vi "FGV.vi"(6 "Dev Type in":T1, 7 "Dev Type Key":string, 8 "error in (no error)":errorcluster, 9 "Device Types in":T1[](array[typedef]), 10 "Action":T6, 11 "Device Type to return":i32=-1) -> (0 "error out":errorcluster, 1 "Dev Types out":T1[](array[typedef]), 2 "found at index":i32, 3 "added?":bool, 4 "Dev Type out":T1)   [LabVIEW 2013, in "daqio minimal.lvlib"]
doc: "This VI is a functional global variable that stores all relevant daq.io account data locally. \n\nKeeping a local device store helps with managing the device data and improves the performance of the overall system. The daq.io LabVIEW API uses this FGV to track and sync required changes that have to be performed online. This FGV should be updated whenever new channels, tags or event types need to generated. The shipping VIs that implicitly auto-create these channels, tags and events make use of this FGV.\n\nTo conserve the amount of transferred data, you can bypass the FGV and use the low level API Call Functions. Then all potential API errors, such as duplicate keys have to be managed on the client side.\n\nSee the \"Connect Device\" function to learn how this FGV can be used."
uses:
  daqio minimal.lvlib
  _typedefs/daqio-Device-Type-Info-return.ctl
  _typedefs/daqio-Channel-Type-POST-return.ctl
  _typedefs/daqio-Device.ctl
  _typedefs/daqio-Event-Type.ctl
  _typedefs/daqio-Tag-Type-POST-return.ctl
  _typedefs/FGV_commands.ctl
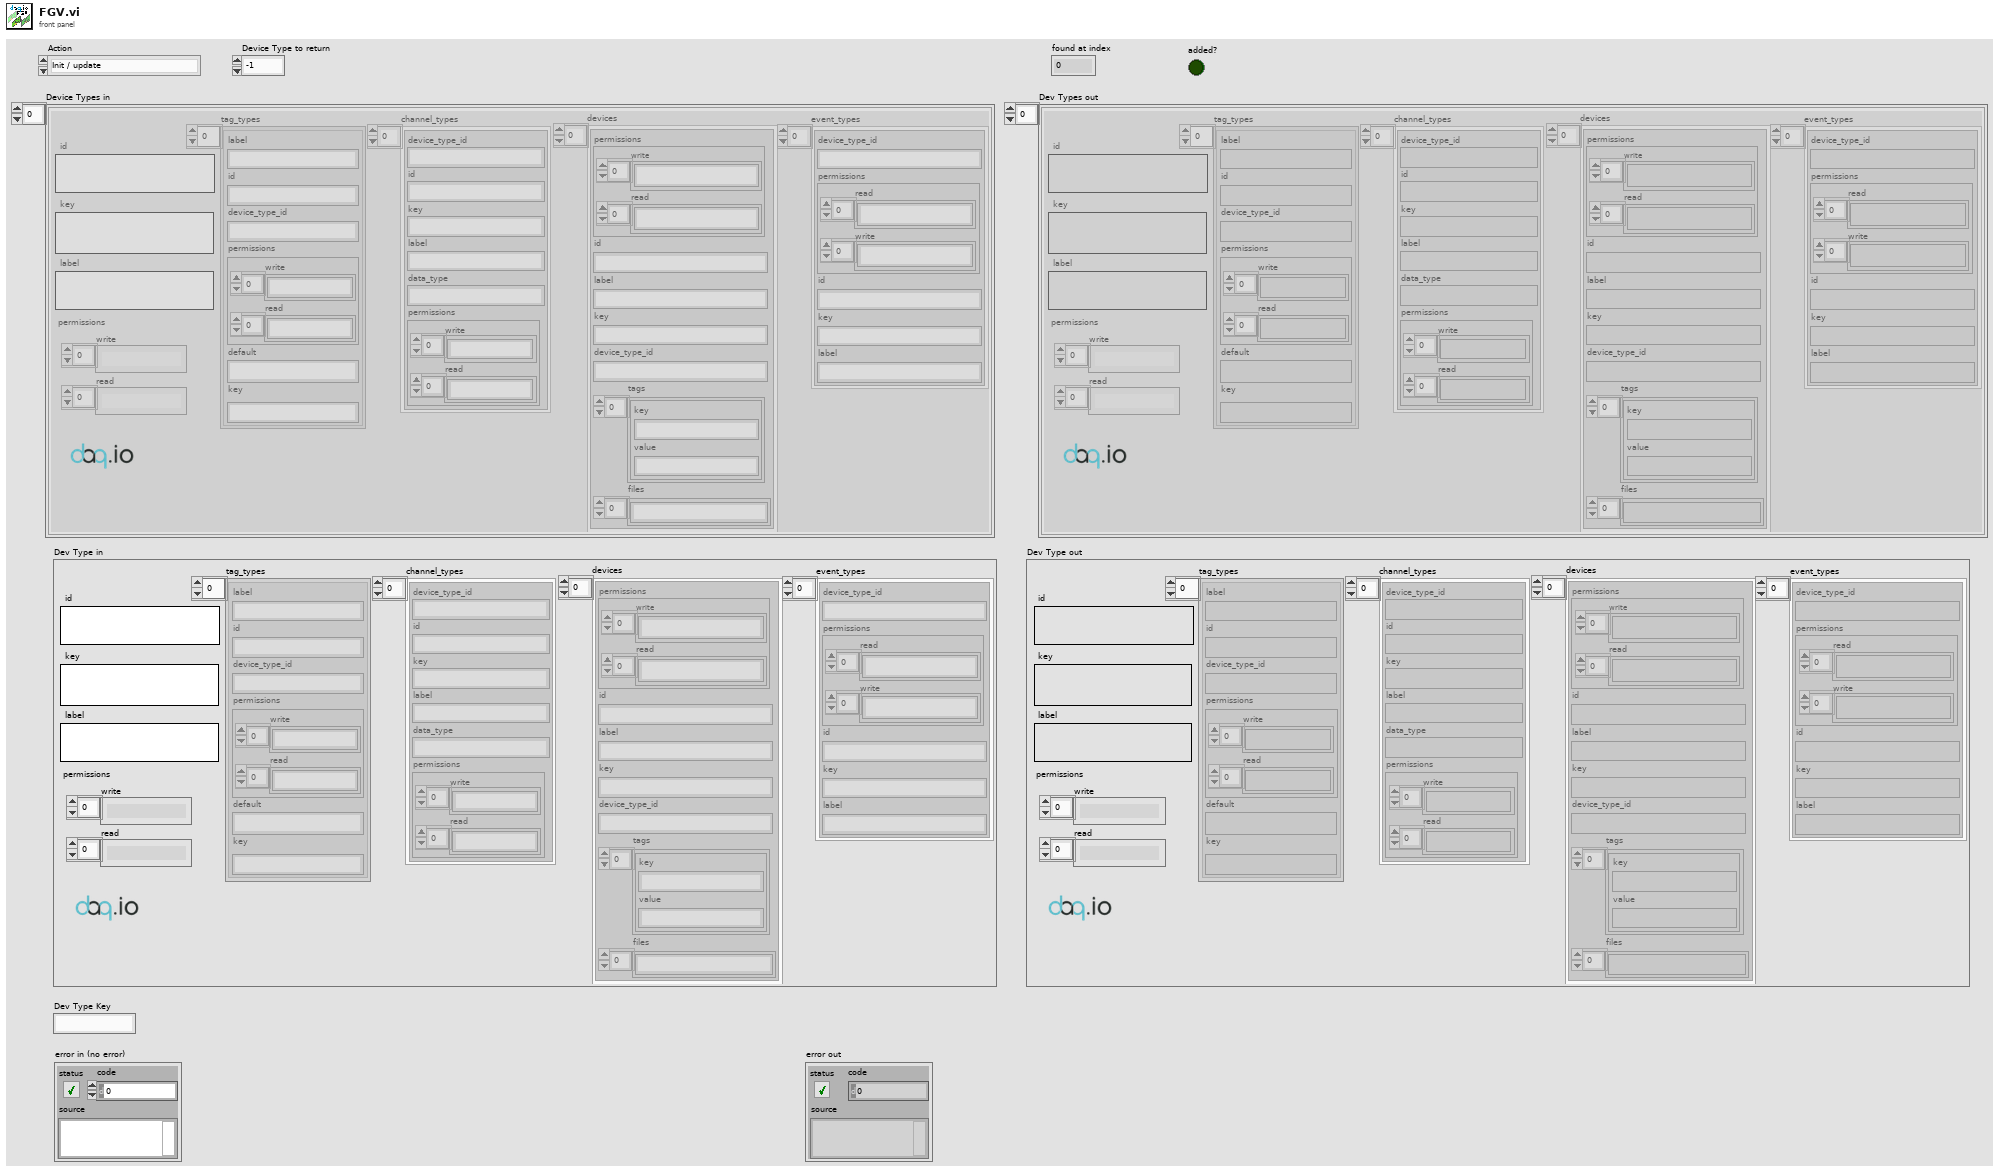
[diagram p1: front panel]
types:
  T1 = typedef "daqio minimal.lvlib/daqio-Device-Type-Info-return.ctl" = cluster{"channel_types":T2[], "devices":T3[], "label":string, "event_types":T4[], "key":string, "tag_types":T5[], "id":string, "permissions":cluster{"write":string[], "read":string[]}}
  T2 = typedef "daqio minimal.lvlib/daqio-Channel-Type-POST-return.ctl" = cluster{"device_type_id":string, "id":string, "key":string, "label":string, "data_type":string, "permissions":cluster{"write":string[], "read":string[]}}
  T3 = typedef "daqio minimal.lvlib/daqio-Device.ctl" = cluster{"permissions":cluster{"write":string[], "read":string[]}, "id":string, "label":string, "key":string, "device_type_id":string, "tags":cluster{"key":string, "value":string}[], "files":string[]}
  T4 = typedef "daqio minimal.lvlib/daqio-Event-Type.ctl" = cluster{"device_type_id":string, "permissions":cluster{"read":string[], "write":string[]}, "id":string, "key":string, "label":string}
  T5 = typedef "daqio minimal.lvlib/daqio-Tag-Type-POST-return.ctl" = cluster{"label":string, "id":string, "device_type_id":string, "permissions":cluster{"write":string[], "read":string[]}, "default":string, "key":string}
  T6 = typedef "daqio minimal.lvlib/FGV_commands.ctl" = enum16{"Init / update", "Edit Item", "Find or Add Item", "Remove Item", "Delete All"}
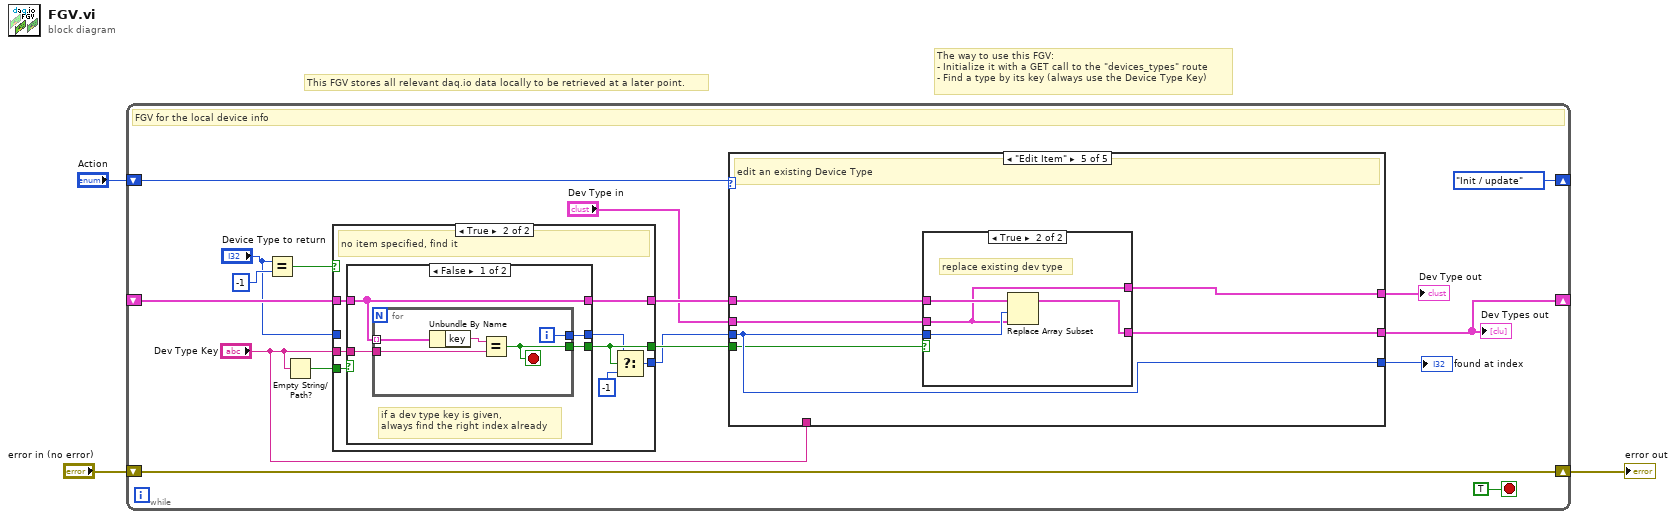
[diagram p0: block diagram]
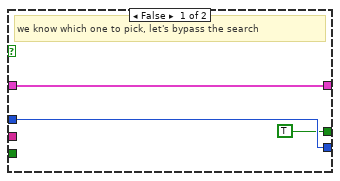
[diagram p2: hidden frame]
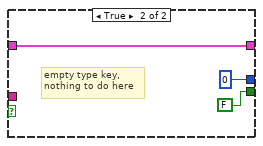
[diagram p3: hidden frame]
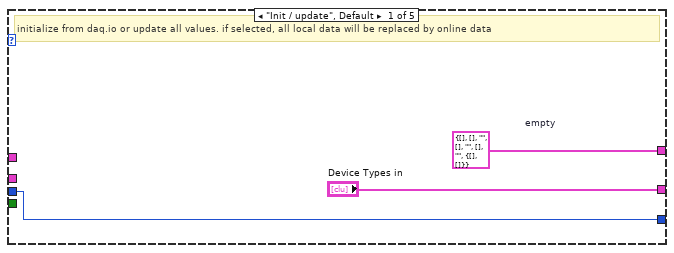
[diagram p4: hidden frame]
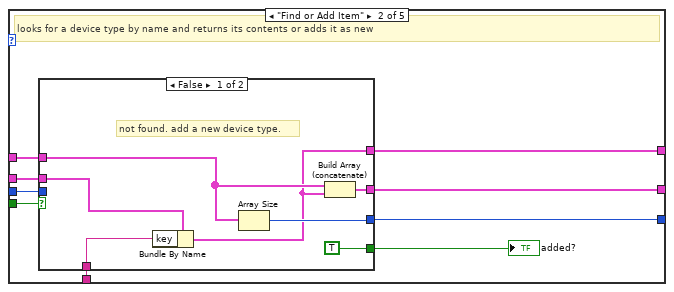
[diagram p5: hidden frame]
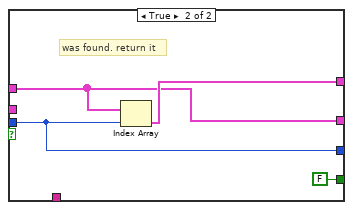
[diagram p6: hidden frame]
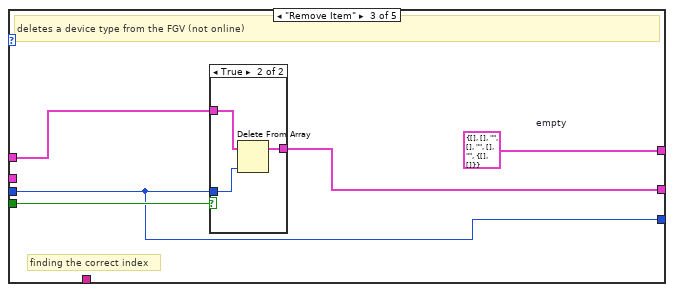
[diagram p7: hidden frame]
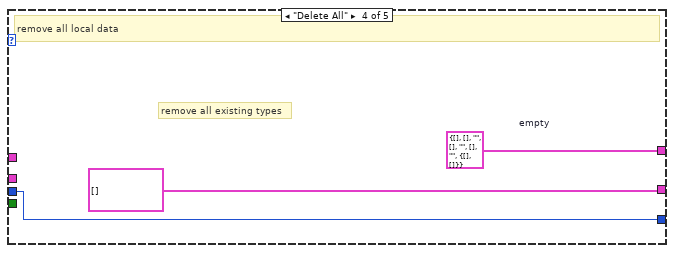
[diagram p9: hidden frame]
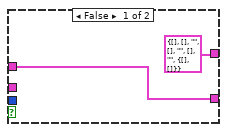
[diagram p10: hidden frame]
diagram:
  # "The way to use this FGV: \n- Initialize it with a GET call to the \"devices_types\" route\n- Find a type by its key (always use the Device Type Key)"
  # "This FGV stores all relevant daq.io data locally to be retrieved at a later point."
  n1 = while {
    shift-right: [FGV_commands."Init / update"] -> _
    shift-left: "Action" -> [w19]
    shift-right: [w18] -> _
    shift-left: _ -> [w14]
    shift-right: [w17] -> w1
    shift-left: "error in (no error)" -> [w17]
    stop <- TRUE stop-if-true
    # "FGV for the local device info"
    n2 = Equal?(x="Device Type to return", y=-1) -> (x = y?=w6:bool)
    n3 = Empty String/Path?(string/path="Dev Type Key") -> (empty?=w15:bool)
    n4 = case shown="True" w6 {
      tunnel: w15 -> [_ w31]
      tunnel: w14 -> [w23 w30]
      tunnel: [w23 w29] -> w13
      tunnel: "Dev Type Key" -> [_ w28]
      tunnel: [TRUE w27] -> w9
      tunnel: [w22 w24] -> w4
      tunnel: "Device Type to return" -> [w22 _]
      frame False {
        # "we know which one to pick, let's bypass the search"
      }
      frame True {
        # "no item specified, find it"
        n5 = case shown="False" w31 {
          tunnel: w30 -> [w35 w43]
          tunnel: [w35 w43] -> w29
          tunnel: w28 -> [w34 _]
          tunnel: [w33 0] -> w26
          tunnel: [w32 FALSE] -> w27
          frame False {
            # "if a dev type key is given, \nalways find the right index already"
            n6 = for {
              tunnel: [w39] -> w33
              tunnel: [w38] -> w32
              tunnel: w35 -> [w37] mode=indexing
              tunnel: w34 -> [w36]
              i -> [w39]
              stop <- w38 stop-if-true
              n7 = Unbundle By Name(w37) -> ("key"=w40:string)
              n8 = Equal?(x=w40, y=w36) -> (x = y?=w38:bool)
            }
          }
          frame True {
            # "empty type key, \nnothing to do here"
          }
        }
        n9 = Select(t=w26, s=w27, f=-1) -> (s? t:f=w24:i32)
      }
    }
    n10 = case shown="\"Edit Item\"" w19 {
      tunnel: ["Device Types in" w55 w70 T1[] [] ("Device Types") w81] -> w18
      tunnel: w13 -> [_ w54 w71 _ w84]
      tunnel: w4 -> [w44 w52 w67 w76 w83]
      tunnel: w9 -> [_ w53 w69 _ w82]
      tunnel: "Dev Type in" -> [_ w50 _ _ w80]
      tunnel: [w45 w51 w68 w77 w79] -> w11
      tunnel: "Dev Type Key" -> [_ w49 _ _ _]
      tunnel: [w44 w47 w67 w76 w83] -> w8
      frame "Init / update", Default {
        w45 = T1 {"channel_types"=[], "devices"=[], "label"="", "event_types"=[], "key"="", "tag_types"=[], "id"="", "permissions"={"write"=[], "read"=[]}}  # empty
        # "initialize from daq.io or update all values. if selected, all local data will be replaced by online data"
      }
      frame "Find or Add Item" {
        # "looks for a device type by name and returns its contents or adds it as new"
        n11 = case shown="False" w53 {
          tunnel: [w62 w65] -> w55
          tunnel: w54 -> [w59 w65]
          tunnel: w52 -> [_ w63]
          tunnel: [w57 w66] -> w51
          tunnel: w50 -> [w61 _]
          tunnel: w49 -> [w60 _]
          tunnel: [w58 w63] -> w47
          tunnel: [TRUE FALSE] -> w48
          frame False {
            # "not found. add a new device type."
            n12 = Bundle By Name(cluster=w61, "key"=w60) -> (w57:T1)
            n13 = Array Size(array=w59) -> (size(s)=w58:i32)
            n14 = Build Array (concatenate)(w59, w57) -> (w62:T1[])
          }
          frame True {
            # "was found. return it"
            n15 = Index Array(array=w65, index=w63) -> (element=w66:T1)
          }
        }
        "added?" <- w48
      }
      frame "Remove Item" {
        w68 = T1 {"channel_types"=[], "devices"=[], "label"="", "event_types"=[], "key"="", "tag_types"=[], "id"="", "permissions"={"write"=[], "read"=[]}}  # empty
        # "finding the correct index"
        # "deletes a device type from the FGV (not online)"
        n16 = case shown="True" w69 {
          tunnel: w71 -> [w72 w75]
          tunnel: [w72 w74] -> w70
          tunnel: w67 -> [_ w73]
          frame False {
          }
          frame True {
            n17 = Delete From Array(array=w75, index=w73) -> (array with subset deleted=w74:T1[])  [unwired: 1 in, 1 out]
          }
        }
      }
      frame "Delete All" {
        w77 = T1 {"channel_types"=[], "devices"=[], "label"="", "event_types"=[], "key"="", "tag_types"=[], "id"="", "permissions"={"write"=[], "read"=[]}}  # empty
        # "remove all existing types"
        # "remove all local data"
      }
      frame "Edit Item" {
        # "edit an existing Device Type"
        n18 = case shown="True" w82 {
          tunnel: w84 -> [w86 w90]
          tunnel: w83 -> [_ w89]
          tunnel: [w86 w88] -> w81
          tunnel: w80 -> [_ w87]
          tunnel: [T1 {"channel_types"=[], "devices"=[], "label"="", "event_types"=[], "key"="", "tag_types"=[], "id"="", "permissions"={"write"=[], "read"=[]}} ("Dev Type in 2") w87] -> w79
          frame False {
          }
          frame True {
            # "replace existing dev type"
            n19 = Replace Array Subset(array=w90, new element=w87, index=w89) -> (w88:T1[])
          }
        }
      }
    }
    "Dev Types out" <- w18
    "Dev Type out" <- w11
    "found at index" <- w8
  }
  "error out" <- w1
